vi "Main WT1600.vi"(0 "Settings WT1600 ing":T3={"data bits"=8, "parity"=0, "stop bits"=10, "flow control"=0, "baud rate"=8, "COM"=""} {"baud rate" min=5 max=8 step=1; "flow control" items=["None"=0, "XON/XOFF"=1, "RTS/CTS"=2, "DTR/DSR"=4]; "stop bits" items=["1.0"=10, "1.5"=15, "2.0"=20]; "parity" items=["None", "Odd", "Even", "Mark", "Space"]; "data bits" min=5 max=8 step=1}, 1 "STOP":bool, 2 "Range Tors.":bool, 3 "Numeric":i64, 4 "WT1600 Config ing 3":T1={"Wiring A (0: 1P2W)"=0, "Wiring B (0: 1P2W)"=0, "Wiring C (0: 1P2W)"=0, "V Range (12: 1000)"=12, "V Element (0: All)"=0, "A Element (0: All)"=0, "A Range (9: 5A)"=9, "A Sensor Ratio(mV/A) (10.0000) "=10.0, "Zero Cross Filter (0: OFF)"=0, "Line Filter (0: OFF)"=0, "PT Ratio (1.0000)"=1.0, "Scaling (F: OFF)"=FALSE, "CT Ratio (1.0000)"=1.0, "Scaling Factor (1.0000)"=1.0, "Filter Element (0: All)"=0, "Display Format (0: Numeric)"=0, "Normal Item Amount (1: 4)"=1, "Harmonics Item Amount (1: 4)"=1, "Average Type (0: OFF)"=0, "Average Count (2: 8)"=2, "A Range (9: 5A) 2"=9, "A Sensor Ratio(mV/A) (10.0000)  2"=10.0, "Zero Cross Filter (0: OFF) 2"=0, "Line Filter (0: OFF) 2"=0, "PT Ratio (1.0000) 2"=1.0, "Scaling (F: OFF) 2"=FALSE, "CT Ratio (1.0000) 2"=1.0, "Scaling Factor (1.0000) 2"=1.0, "CUT OFF FREQ"=0.0} {"Wiring A (0: 1P2W)" items=["1P2W", "1P3W", "3P3W", "3P4W", "3V3A"]; "Wiring B (0: 1P2W)" items=["1P2W", "1P3W", "3P3W", "3P4W", "3V3A", "NONE"]; "Wiring C (0: 1P2W)" items=["1P2W", "1P3W", "3P3W", "3P4W", "3V3A", "NONE"]; "V Range (12: 1000)" items=["AUTO", "1.5", "3", "6", "10", "15", "30", "60", "100", "150", "300", "600", "1000"]; "V Element (0: All)" items=["All", "Element 1", "Element 2", "Element 3", "Element 4", "Element 5", "Element 6"]; "A Element (0: All)" items=["All", "Element 1", "Element 2", "Element 3", "Element 4", "Element 5", "Element 6"]; "A Range (9: 5A)" items=["AUTO", "10 mA", "20 mA", "50 mA", "100 mA", "200 mA", "500 mA", "1 A", "2 A", "5 A", "10 A", "20 A", "50 A", "S-AUTO", "50 mV", "100 mV", "250 mV", "500 mV", "1 V", "2.5 V", "5 V", "10 V"]; "Zero Cross Filter (0: OFF)" items=["OFF", "500Hz"]; "Line Filter (0: OFF)" items=["OFF", "500Hz", "5.5kHz"]; "Filter Element (0: All)" items=["All", "Element 1", "Element 2", "Element 3", "Element 4", "Element 5", "Element 6"]; "Display Format (0: Numeric)" items=["Numeric", "Wave", "Bar", "Vector", "Trend", "Numeric & Wave", "Numeric & Bar", "Numeric & Trend", "Wave & Bar", "Wave & Trend", "Bar & Trend", "Information"]; "Normal Item Amount (1: 4)" items=["ALL", "4", "8", "16", "42", "78"]; "Harmonics Item Amount (1: 4)" items=["-", "4", "8", "16", "Single List", "Dual List", "Sigma List"]; "Average Type (0: OFF)" items=["OFF", "Linear", "Exponent"]; "Average Count (2: 8)" items=["2", "4", "8", "16", "32", "64", "128", "256"]; "A Range (9: 5A) 2" items=["AUTO", "10 mA", "20 mA", "50 mA", "100 mA", "200 mA", "500 mA", "1 A", "2 A", "5 A", "10 A", "20 A", "50 A", "S-AUTO", "50 mV", "100 mV", "250 mV", "500 mV", "1 V", "2.5 V", "5 V", "10 V"]; "Zero Cross Filter (0: OFF) 2" items=["OFF", "500Hz"]; "Line Filter (0: OFF) 2" items=["OFF", "500Hz", "5.5kHz"]}, 5 "Refresh":bool, 7 "Path":string) -> (9 "error out":errorcluster, 10 "WT1600 Config ing":T1={"Wiring A (0: 1P2W)"=0, "Wiring B (0: 1P2W)"=0, "Wiring C (0: 1P2W)"=0, "V Range (12: 1000)"=12, "V Element (0: All)"=0, "A Element (0: All)"=0, "A Range (9: 5A)"=9, "A Sensor Ratio(mV/A) (10.0000) "=10.0, "Zero Cross Filter (0: OFF)"=0, "Line Filter (0: OFF)"=0, "PT Ratio (1.0000)"=1.0, "Scaling (F: OFF)"=FALSE, "CT Ratio (1.0000)"=1.0, "Scaling Factor (1.0000)"=1.0, "Filter Element (0: All)"=0, "Display Format (0: Numeric)"=0, "Normal Item Amount (1: 4)"=1, "Harmonics Item Amount (1: 4)"=1, "Average Type (0: OFF)"=0, "Average Count (2: 8)"=2, "A Range (9: 5A) 2"=9, "A Sensor Ratio(mV/A) (10.0000)  2"=10.0, "Zero Cross Filter (0: OFF) 2"=0, "Line Filter (0: OFF) 2"=0, "PT Ratio (1.0000) 2"=1.0, "Scaling (F: OFF) 2"=FALSE, "CT Ratio (1.0000) 2"=1.0, "Scaling Factor (1.0000) 2"=1.0, "CUT OFF FREQ"=0.0} {"Wiring A (0: 1P2W)" items=["1P2W", "1P3W", "3P3W", "3P4W", "3V3A"]; "Wiring B (0: 1P2W)" items=["1P2W", "1P3W", "3P3W", "3P4W", "3V3A", "NONE"]; "Wiring C (0: 1P2W)" items=["1P2W", "1P3W", "3P3W", "3P4W", "3V3A", "NONE"]; "V Range (12: 1000)" items=["AUTO", "1.5", "3", "6", "10", "15", "30", "60", "100", "150", "300", "600", "1000"]; "V Element (0: All)" items=["All", "Element 1", "Element 2", "Element 3", "Element 4", "Element 5", "Element 6"]; "A Element (0: All)" items=["All", "Element 1", "Element 2", "Element 3", "Element 4", "Element 5", "Element 6"]; "A Range (9: 5A)" items=["AUTO", "10 mA", "20 mA", "50 mA", "100 mA", "200 mA", "500 mA", "1 A", "2 A", "5 A", "10 A", "20 A", "50 A", "S-AUTO", "50 mV", "100 mV", "250 mV", "500 mV", "1 V", "2.5 V", "5 V", "10 V"]; "Zero Cross Filter (0: OFF)" items=["OFF", "500Hz"]; "Line Filter (0: OFF)" items=["OFF", "500Hz", "5.5kHz"]; "Filter Element (0: All)" items=["All", "Element 1", "Element 2", "Element 3", "Element 4", "Element 5", "Element 6"]; "Display Format (0: Numeric)" items=["Numeric", "Wave", "Bar", "Vector", "Trend", "Numeric & Wave", "Numeric & Bar", "Numeric & Trend", "Wave & Bar", "Wave & Trend", "Bar & Trend", "Information"]; "Normal Item Amount (1: 4)" items=["ALL", "4", "8", "16", "42", "78"]; "Harmonics Item Amount (1: 4)" items=["-", "4", "8", "16", "Single List", "Dual List", "Sigma List"]; "Average Type (0: OFF)" items=["OFF", "Linear", "Exponent"]; "Average Count (2: 8)" items=["2", "4", "8", "16", "32", "64", "128", "256"]; "A Range (9: 5A) 2" items=["AUTO", "10 mA", "20 mA", "50 mA", "100 mA", "200 mA", "500 mA", "1 A", "2 A", "5 A", "10 A", "20 A", "50 A", "S-AUTO", "50 mV", "100 mV", "250 mV", "500 mV", "1 V", "2.5 V", "5 V", "10 V"]; "Zero Cross Filter (0: OFF) 2" items=["OFF", "500Hz"]; "Line Filter (0: OFF) 2" items=["OFF", "500Hz", "5.5kHz"]}, 11 "error out 2":errorcluster, 12 "Cluster wt1600":T2, 14 "Settings WT1600 out":T3={"data bits"=8, "parity"=0, "stop bits"=10, "flow control"=0, "baud rate"=8, "COM"=""} {"baud rate" min=5 max=8 step=1; "flow control" items=["None"=0, "XON/XOFF"=1, "RTS/CTS"=2, "DTR/DSR"=4]; "stop bits" items=["1.0"=10, "1.5"=15, "2.0"=20]; "parity" items=["None", "Odd", "Even", "Mark", "Space"]; "data bits" min=5 max=8 step=1}, 15 "WT1600":bool, 16 "Errori WT1600":i64, 17 "Measure Value":sgl[](array[numeric]) format="%^.3e", 18 "Coppia":dbl, 19 "Velocità":dbl)   [LabVIEW 2016]
uses:
  QSM PC EXAMPLE.llb/wt1600 variabili.ctl
panel:
  in  "termination char\n(0xA = '\\n' = LF)":u8=10 format="%.0x"
  in  "MaxErr WT1600":i64
  # "ON\nOFF"
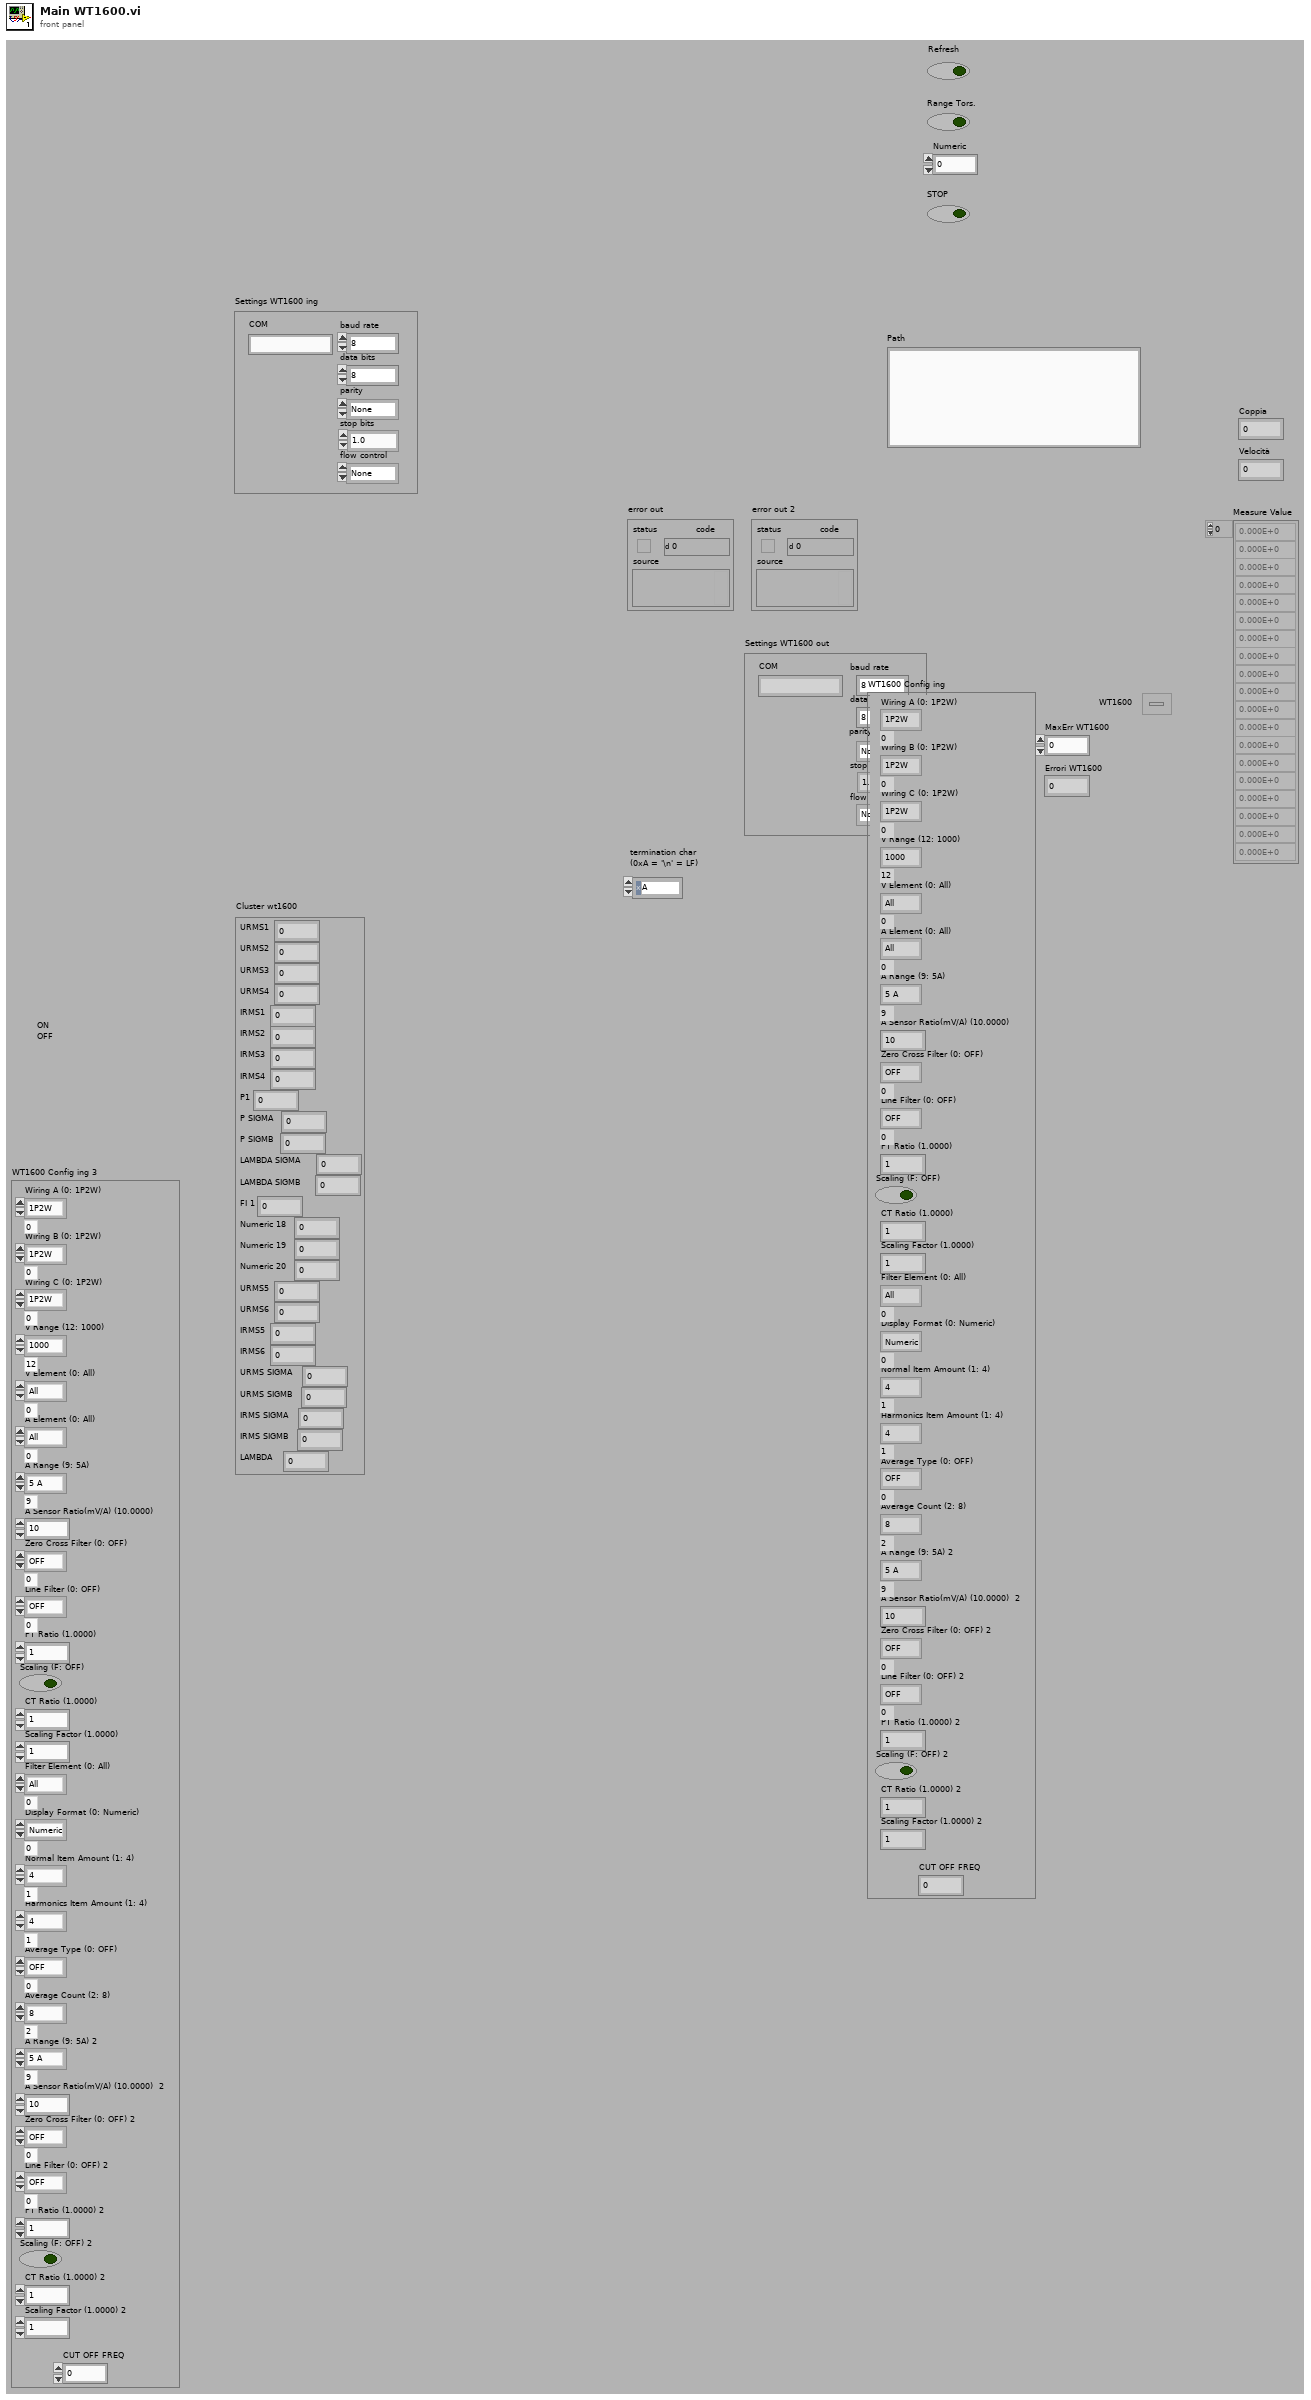
[diagram p1: front panel]
types:
  T1 = cluster{"Wiring A (0: 1P2W)":u16, "Wiring B (0: 1P2W)":u16, "Wiring C (0: 1P2W)":u16, "V Range (12: 1000)":u16, "V Element (0: All)":u16, "A Element (0: All)":u16, "A Range (9: 5A)":u16, "A Sensor Ratio(mV/A) (10.0000) ":dbl, "Zero Cross Filter (0: OFF)":u16, "Line Filter (0: OFF)":u16, "PT Ratio (1.0000)":dbl, "Scaling (F: OFF)":bool, "CT Ratio (1.0000)":dbl, "Scaling Factor (1.0000)":dbl, "Filter Element (0: All)":u16, "Display Format (0: Numeric)":u16, "Normal Item Amount (1: 4)":u16, "Harmonics Item Amount (1: 4)":u16, "Average Type (0: OFF)":u16, "Average Count (2: 8)":u16, "A Range (9: 5A) 2":u16, "A Sensor Ratio(mV/A) (10.0000)  2":dbl, "Zero Cross Filter (0: OFF) 2":u16, "Line Filter (0: OFF) 2":u16, "PT Ratio (1.0000) 2":dbl, "Scaling (F: OFF) 2":bool, "CT Ratio (1.0000) 2":dbl, "Scaling Factor (1.0000) 2":dbl, "CUT OFF FREQ":dbl}
  T2 = typedef "wt1600 variabili.ctl" = cluster{"URMS1":dbl, "URMS2":dbl, "URMS3":dbl, "URMS4":dbl, "IRMS1":dbl, "IRMS2":dbl, "IRMS3":dbl, "IRMS4":dbl, "P1":dbl, "P SIGMA":dbl, "P SIGMB":dbl, "LAMBDA SIGMA":dbl, "LAMBDA SIGMB":dbl, "FI 1":dbl, "Numeric 18":dbl, "Numeric 19":dbl, "Numeric 20":dbl, "URMS5":dbl, "URMS6":dbl, "IRMS5":dbl, "IRMS6":dbl, "URMS SIGMA":dbl, "URMS SIGMB":dbl, "IRMS SIGMA":dbl, "IRMS SIGMB":dbl, "LAMBDA":dbl}
  T3 = cluster{"data bits":u16, "parity":u16, "stop bits":u16, "flow control":u16, "baud rate":u16, "COM":string}
  T4 = cluster{"URMS1":dbl, "URMS2":dbl, "URMS3":dbl, "URMS4":dbl, "IRMS1":dbl, "IRMS2":dbl, "IRMS3":dbl, "IRMS4":dbl, "P1":dbl, "P SIGMA":dbl, "P SIGMB":dbl, "LAMBDA SIGMA":dbl, "LAMBDA SIGMB":dbl, "FI 1":dbl, "Numeric 18":dbl, "Numeric 19":dbl, "Numeric 20":dbl, "URMS5":dbl, "URMS6":dbl, "IRMS5":dbl, "IRMS6":dbl, "URMS SIGMA":dbl, "URMS SIGMB":dbl, "IRMS SIGMA":dbl, "IRMS SIGMB":dbl, "LAMBDA":dbl}
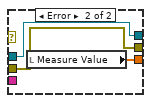
[diagram p4: hidden frame]
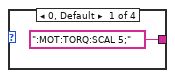
[diagram p6: hidden frame]
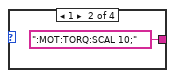
[diagram p7: hidden frame]
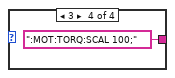
[diagram p8: hidden frame]
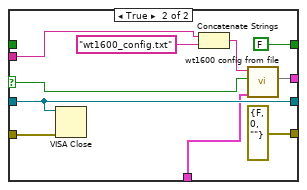
[diagram p10: hidden frame]
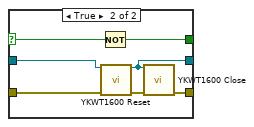
[diagram p13: hidden frame]
diagram:
  n1 = flat-sequence {
    tunnel: [w2] -> w1
    tunnel: w1 -> [w14]
    frame #0 {
      n2 = flat-sequence {
        frame #0 {
        }
      }
      n3 = flat-sequence {
        tunnel: ["Path"] -> w2
        frame #0 {
          n4 = First Call?() -> (First Call?: T/F=w6:bool)
          n5 = case shown="True" w6 {
            tunnel: [w7 w10] -> w4
            tunnel: "Settings WT1600 ing" -> [w7 w11]
            tunnel: "Path" -> [_ w8]
            frame False {
            }
            frame True {
              n6 = local write "MaxErr WT1600"(10) -> ()
              n7 = Concatenate Strings(w8, "wt1600.txt") -> (w12:string)
              n8 = call "Read config COM.vi"("Path"=w12, "Settings WT1600 ing"=w11) -> ("Settings WT1600 out"=w10:T3)  [unwired: 9 out]
            }
          }
          "Settings WT1600 out" <- w4
        }
      }
    }
    frame #1 {
      n9 = while {
        shift-right: [w25] -> _
        shift-left: _ -> [w26]
        shift-right: [w18] -> _
        shift-left: _ -> [w24]
        shift-right: [w19] -> _
        shift-left: _ -> [w27]
        tunnel: w14 -> [w20]
        stop <- TRUE stop-if-true
        n10 = Not(x="STOP") -> (.not. x?=w23:bool)
        n11 = case shown="True" w23 {
          tunnel: w27 -> [_ w81]
          tunnel: w26 -> [w30 w83]
          tunnel: [w30 w91] -> w25
          tunnel: [w31 w90] -> w18
          tunnel: w24 -> [w31 w82]
          tunnel: [FALSE w89] -> w19
          tunnel: w20 -> [_ w72]
          tunnel: [errorcluster {"status"=TRUE, "code"=0, "source"=""} ("´×°oÍ") w34] -> w15
          frame False {
          }
          frame True {
            (unwired) ":NUM:NORM:NUM 8;ITEM1 URMS,SIGMA;ITEM2 IRMS,SIGMA;ITEM3 LAMBDA,SIGMA;ITEM4 FU,1;ITEM5 P,SIGMA;ITEM6 S,SIGMA;ITEM7 Q,SIGMA;ITEM8 IRMS,1; VAL?;"
            # "URMS1\nURMS2\nURMS3\nURMS4\nURMS5\nURMS6\nURMS SIGMA\nURMS SIGMB\nIRMS1\nIRMS2\nIRMS3\nIRMS4\nIRMS5\nIRMS6\nIRMS SIGMA\nIRMS SIGMB\nP1\nP SIGMA\nP SIGMB\nLAMBDA\nLAMBDA SIGMA\nLAMBDA SIGMB\nFI 1"
            n12 = First Call?() -> (First Call?: T/F=w75:bool)
            n13 = Compound Arithmetic op=OR("Refresh", w75) -> (w74:bool)
            n14 = case shown="False" w74 {
              selector: w74 -> [_ w140]
              tunnel: [w134 w145] -> w80
              tunnel: w83 -> [w134 w145]
              tunnel: [w135 errorcluster {"status"=FALSE, "code"=0, "source"=""} ("error out")] -> w79
              tunnel: w82 -> [w135 w144]
              tunnel: [w136 FALSE] -> w78
              tunnel: w81 -> [w136 _]
              tunnel: w72 -> [_ w141]
              tunnel: [w133 w138] -> w33
              tunnel: "WT1600 Config ing 3" -> [w133 w137]
              frame False {
              }
              frame True {
                n15 = VISA Close(VISA resource name=w145, error in (no error)=w144) -> ()  [unwired: 1 out]
                n16 = Concatenate Strings(w141, "wt1600_config.txt") -> (w142:string)
                n17 = call "wt1600 config from file.vi"("WT1600 Config ing"=w137, "leggi"=w140, "Path"=w142) -> (2:w138)  [unwired: 1 in, 7 out]
              }
            }
            "WT1600 Config ing" <- w33
            n18 = case shown="False" w78 {
              tunnel: [w153 w324] -> w71
              tunnel: [w152 w325] -> w35
              tunnel: w79 -> [_ w325]
              tunnel: w80 -> [_ w324]
              tunnel: w33 -> [w155 _]
              frame False {
                w148 = TRUE
                n19 = flat-sequence {
                  tunnel: [TRUE] -> w164
                  tunnel: ["termination char\n(0xA = '\\n' = LF)"] -> w163
                  tunnel: [50] -> w162
                  frame #0 {
                  }
                }
                n20 = local read "Settings WT1600 out"() -> (w161:T3)
                n21 = Unbundle By Name(w161) -> ("COM"=w154:string, "baud rate"=w160:u16, "data bits"=w159:u16, "stop bits"=w158:u16, "flow control"=w156:u16, "parity"=w157:u16)
                n22 = call "OpenCOM.vi"("VISA resource name"=w154, "baud rate (9600)"=w160, "data bits"=w159, "parity"=w157, "stop bits"=w158, "flow control"=w156, "termination char\n(0xA = '\\n' = LF)"=w163, "timeout(ms) solitamente 50ms"=w162, "End Write termination character?"=w164, "End read on termination character?"=w164) -> ("VISA resource name out"=w151:refnum<visa-resource-name>, "error out"=w150:errorcluster)  [unwired: 16 out]
                n23 = call "YKWT1600 Initialize.vi"("VISA session (for class)"=w151, "ID Query (T: Check)"=w148, "Reset (T: Reset)"=w148, "error in (no error)"=w150) -> ("VISA session"=w149:refnum<visa-resource-name>, "error out"=w147:errorcluster)  [unwired: 10 out]
                n24 = case shown="No Error" w147 {
                  tunnel: w155 -> [w167 _]
                  tunnel: w147 -> [w233 w320]
                  tunnel: w149 -> [w232 w319]
                  tunnel: [w230 w319] -> w153
                  tunnel: [w229 w320] -> w152
                  frame No Error {
                    w181 = u16 6 items=["All", "Element 1", "Element 2", "Element 3", "Element 4", "Element 5", "Element 6"] ("Element (0: All)")
                    w180 = u16 5 items=["All", "Element 1", "Element 2", "Element 3", "Element 4", "Element 5", "Element 6"] ("Element (0: All)")
                    w179 = u16 4 items=["All", "Element 1", "Element 2", "Element 3", "Element 4", "Element 5", "Element 6"] ("Element (0: All)")
                    w177 = u16 3 items=["All", "Element 1", "Element 2", "Element 3", "Element 4", "Element 5", "Element 6"] ("Element (0: All)")
                    w178 = u16 2 items=["All", "Element 1", "Element 2", "Element 3", "Element 4", "Element 5", "Element 6"] ("Element (0: All)")
                    w176 = u16 1 items=["All", "Element 1", "Element 2", "Element 3", "Element 4", "Element 5", "Element 6"] ("Element (0: All)")
                    w207 = u16 6 items=["All", "Element 1", "Element 2", "Element 3", "Element 4", "Element 5", "Element 6"] ("Element (0: All)")
                    w208 = u16 5 items=["All", "Element 1", "Element 2", "Element 3", "Element 4", "Element 5", "Element 6"] ("Element (0: All)")
                    w209 = u16 4 items=["All", "Element 1", "Element 2", "Element 3", "Element 4", "Element 5", "Element 6"] ("Element (0: All)")
                    w210 = u16 3 items=["All", "Element 1", "Element 2", "Element 3", "Element 4", "Element 5", "Element 6"] ("Element (0: All)")
                    w206 = u16 2 items=["All", "Element 1", "Element 2", "Element 3", "Element 4", "Element 5", "Element 6"] ("Element (0: All)")
                    w211 = u16 1 items=["All", "Element 1", "Element 2", "Element 3", "Element 4", "Element 5", "Element 6"] ("Element (0: All)")
                    w245 = u16 1 items=["50ms", "100ms", "200ms", "500ms", "1s", "2s", "5s"] ("Update Rate (3: 500ms)")
                    n25 = Unbundle By Name(w167) -> ("Wiring A (0: 1P2W)"=w258:u16, "Wiring B (0: 1P2W)"=w257:u16, "Wiring C (0: 1P2W)"=w256:u16, "V Range (12: 1000)"=w266:u16, "V Element (0: All)"=w265:u16, "A Range (9: 5A)"=w175:u16, "A Sensor Ratio(mV/A) (10.0000)"=w174:dbl, "Zero Cross Filter (0: OFF)"=w203:u16, "Line Filter (0: OFF)"=w204:u16, "PT Ratio (1.0000)"=w202:dbl, "Scaling (F: OFF)"=w205:bool, "CT Ratio (1.0000)"=w201:dbl, "Scaling Factor (1.0000)"=w200:dbl, "Display Format (0: Numeric)"=w264:u16, "Normal Item Amount (1: 4)"=w263:u16, "Harmonics Item Amount (1: 4)"=w262:u16, "Average Type (0: OFF)"=w260:u16, "Average Count (2: 8)"=w259:u16)  [unwired: 2 out]
                    n26 = call "YKWT1600 Config Filter & Scaling.vi"("VISA session"=w232, "Scaling (F: OFF)"=w205, "Element (0: All)"=w211, "Line Filter (0: OFF)"=w204, "WT 1600 Zero Cross Filter (0: OFF)"=w203, "error in (no error)"=w233, "PT Ratio (1.0000)"=w202, "CT Ratio (1.0000)"=w201, "Scaling Factor (1.0000)"=w200) -> ("dup VISA session"=w228:refnum<visa-resource-name>, "error out"=w231:errorcluster)  [unwired: 2 in, 3 out]
                    n27 = flat-sequence {
                      tunnel: w231 -> [w305]
                      tunnel: [w305] -> w227
                      frame #0 {
                        n28 = Wait (ms)(milliseconds to wait=2000) -> ()  [unwired: 1 out]
                      }
                    }
                    n29 = call "YKWT1600 Config Filter & Scaling.vi"("VISA session"=w228, "Scaling (F: OFF)"=w205, "Element (0: All)"=w206, "Line Filter (0: OFF)"=w204, "WT 1600 Zero Cross Filter (0: OFF)"=w203, "error in (no error)"=w227, "PT Ratio (1.0000)"=w202, "CT Ratio (1.0000)"=w201, "Scaling Factor (1.0000)"=w200) -> ("dup VISA session"=w213:refnum<visa-resource-name>, "error out"=w226:errorcluster)  [unwired: 2 in, 3 out]
                    n30 = flat-sequence {
                      tunnel: w226 -> [w303]
                      tunnel: [w303] -> w225
                      frame #0 {
                        n31 = Wait (ms)(milliseconds to wait=2000) -> ()  [unwired: 1 out]
                      }
                    }
                    n32 = call "YKWT1600 Config Filter & Scaling.vi"("VISA session"=w213, "Scaling (F: OFF)"=w205, "Element (0: All)"=w210, "Line Filter (0: OFF)"=w204, "WT 1600 Zero Cross Filter (0: OFF)"=w203, "error in (no error)"=w225, "PT Ratio (1.0000)"=w202, "CT Ratio (1.0000)"=w201, "Scaling Factor (1.0000)"=w200) -> ("dup VISA session"=w216:refnum<visa-resource-name>, "error out"=w224:errorcluster)  [unwired: 2 in, 3 out]
                    n33 = flat-sequence {
                      tunnel: [w300] -> _
                      tunnel: [w300] -> w223
                      tunnel: w224 -> [w300]
                      frame #0 {
                        n34 = Wait (ms)(milliseconds to wait=2000) -> ()  [unwired: 1 out]
                      }
                    }
                    n35 = Unbundle By Name(w167) -> ("Line Filter (0: OFF) 2"=w173:u16, "Zero Cross Filter (0: OFF) 2"=w172:u16, "Scaling (F: OFF) 2"=w171:bool, "PT Ratio (1.0000) 2"=w170:dbl, "CT Ratio (1.0000) 2"=w169:dbl, "Scaling Factor (1.0000) 2"=w168:dbl)
                    n36 = call "YKWT1600 Config Filter & Scaling.vi"("VISA session"=w216, "Scaling (F: OFF)"=w171, "Element (0: All)"=w209, "Line Filter (0: OFF)"=w173, "WT 1600 Zero Cross Filter (0: OFF)"=w172, "error in (no error)"=w223, "PT Ratio (1.0000)"=w170, "CT Ratio (1.0000)"=w169, "Scaling Factor (1.0000)"=w168) -> ("dup VISA session"=w215:refnum<visa-resource-name>, "error out"=w222:errorcluster)  [unwired: 2 in, 3 out]
                    n37 = flat-sequence {
                      tunnel: w222 -> [w299]
                      tunnel: [w299] -> w221
                      frame #0 {
                        n38 = Wait (ms)(milliseconds to wait=2000) -> ()  [unwired: 1 out]
                      }
                    }
                    n39 = call "YKWT1600 Config Filter & Scaling.vi"("VISA session"=w215, "Scaling (F: OFF)"=w171, "Element (0: All)"=w208, "Line Filter (0: OFF)"=w173, "WT 1600 Zero Cross Filter (0: OFF)"=w172, "error in (no error)"=w221, "PT Ratio (1.0000)"=w170, "CT Ratio (1.0000)"=w169, "Scaling Factor (1.0000)"=w168) -> ("dup VISA session"=w214:refnum<visa-resource-name>, "error out"=w220:errorcluster)  [unwired: 2 in, 3 out]
                    n40 = flat-sequence {
                      tunnel: w220 -> [w297]
                      tunnel: [w297] -> w219
                      frame #0 {
                        n41 = Wait (ms)(milliseconds to wait=2000) -> ()  [unwired: 1 out]
                      }
                    }
                    n42 = call "YKWT1600 Config Filter & Scaling.vi"("VISA session"=w214, "Scaling (F: OFF)"=w171, "Element (0: All)"=w207, "Line Filter (0: OFF)"=w173, "WT 1600 Zero Cross Filter (0: OFF)"=w172, "error in (no error)"=w219, "PT Ratio (1.0000)"=w170, "CT Ratio (1.0000)"=w169, "Scaling Factor (1.0000)"=w168) -> ("dup VISA session"=w212:refnum<visa-resource-name>, "error out"=w218:errorcluster)  [unwired: 2 in, 3 out]
                    n43 = flat-sequence {
                      tunnel: w218 -> [w295]
                      tunnel: [w295] -> w217
                      frame #0 {
                        n44 = Wait (ms)(milliseconds to wait=2000) -> ()  [unwired: 1 out]
                      }
                    }
                    n45 = call "YKWT1600 Config Voltage.vi"("VISA session"=w212, "Element (0: All)"=w265, "V Range (12: 1000)"=w266, "error in (no error)"=w217) -> ("dup VISA session"=w268:refnum<visa-resource-name>, "error out"=w267:errorcluster)  [unwired: 10 out]
                    n46 = call "YKWT1600 Config Current.vi"("VISA session"=w268, "Element (0: All)"=w176, "A Range (9: 5A)"=w175, 9:w174, "error in (no error)"=w267) -> ("dup VISA session"=w183:refnum<visa-resource-name>, "error out"=w189:errorcluster)  [unwired: 9 out]
                    n47 = flat-sequence {
                      tunnel: w189 -> [w293]
                      tunnel: [w293] -> w199
                      frame #0 {
                        n48 = Wait (ms)(milliseconds to wait=2000) -> ()  [unwired: 1 out]
                      }
                    }
                    n49 = call "YKWT1600 Config Current.vi"("VISA session"=w183, "Element (0: All)"=w178, "A Range (9: 5A)"=w175, 9:w174, "error in (no error)"=w199) -> ("dup VISA session"=w187:refnum<visa-resource-name>, "error out"=w198:errorcluster)  [unwired: 9 out]
                    n50 = flat-sequence {
                      tunnel: w198 -> [w291]
                      tunnel: [w291] -> w197
                      frame #0 {
                        n51 = Wait (ms)(milliseconds to wait=2000) -> ()  [unwired: 1 out]
                      }
                    }
                    n52 = call "YKWT1600 Config Current.vi"("VISA session"=w187, "Element (0: All)"=w177, "A Range (9: 5A)"=w175, 9:w174, "error in (no error)"=w197) -> ("dup VISA session"=w186:refnum<visa-resource-name>, "error out"=w196:errorcluster)  [unwired: 9 out]
                    n53 = flat-sequence {
                      tunnel: w196 -> [w289]
                      tunnel: [w289] -> w195
                      frame #0 {
                        n54 = Wait (ms)(milliseconds to wait=2000) -> ()  [unwired: 1 out]
                      }
                    }
                    n55 = Unbundle By Name(w167) -> ("A Range (9: 5A) 2"=w166:u16, "A Sensor Ratio(mV/A) (10.0000)  2"=w165:dbl)
                    n56 = call "YKWT1600 Config Current.vi"("VISA session"=w186, "Element (0: All)"=w179, "A Range (9: 5A)"=w166, 9:w165, "error in (no error)"=w195) -> ("dup VISA session"=w185:refnum<visa-resource-name>, "error out"=w194:errorcluster)  [unwired: 9 out]
                    n57 = flat-sequence {
                      tunnel: w194 -> [w287]
                      tunnel: [w287] -> w193
                      frame #0 {
                        n58 = Wait (ms)(milliseconds to wait=2000) -> ()  [unwired: 1 out]
                      }
                    }
                    n59 = call "YKWT1600 Config Current.vi"("VISA session"=w185, "Element (0: All)"=w180, "A Range (9: 5A)"=w166, 9:w165, "error in (no error)"=w193) -> ("dup VISA session"=w184:refnum<visa-resource-name>, "error out"=w192:errorcluster)  [unwired: 9 out]
                    n60 = flat-sequence {
                      tunnel: [w284] -> w191
                      tunnel: w192 -> [w284]
                      frame #0 {
                        n61 = Wait (ms)(milliseconds to wait=2000) -> ()  [unwired: 1 out]
                      }
                    }
                    n62 = call "YKWT1600 Config Current.vi"("VISA session"=w184, "Element (0: All)"=w181, "A Range (9: 5A)"=w166, 9:w165, "error in (no error)"=w191) -> ("dup VISA session"=w182:refnum<visa-resource-name>, "error out"=w190:errorcluster)  [unwired: 9 out]
                    n63 = flat-sequence {
                      tunnel: [w282] -> w188
                      tunnel: w190 -> [w282]
                      frame #0 {
                        n64 = Wait (ms)(milliseconds to wait=2000) -> ()  [unwired: 1 out]
                      }
                    }
                    n65 = call "YKWT1600 Config Display Format.vi"("VISA session"=w182, "Display Format (0: Numeric)"=w264, "Normal Item Amount (1: 4)"=w263, "Harmonics Item Amount (1: 4)"=w262, "error in (no error)"=w188) -> ("dup VISA session"=w249:refnum<visa-resource-name>, "error out"=w250:errorcluster)  [unwired: 9 out]
                    n66 = flat-sequence {
                      tunnel: w250 -> [w316]
                      tunnel: [w316] -> w247
                      frame #0 {
                        n67 = Wait (ms)(milliseconds to wait=2000) -> ()  [unwired: 1 out]
                      }
                    }
                    n68 = call "YKWT1600 Config Update Rate.vi"("VISA session"=w249, "Update Rate (3: 500ms)"=w245, "error in (no error)"=w247) -> ("dup VISA session"=w248:refnum<visa-resource-name>, "error out"=w246:errorcluster)  [unwired: 11 out]
                    n69 = flat-sequence {
                      tunnel: [w274] -> w261
                      tunnel: [w275] -> w235
                      tunnel: w248 -> [w273]
                      tunnel: w246 -> [w272]
                      tunnel: w256 -> [w269]
                      tunnel: w257 -> [w270]
                      tunnel: w258 -> [w271]
                      frame #0 {
                        n70 = call "YKWT1600 Config Wiring.vi"("VISA session"=w273, "Wiring A (0: 1P2W)"=w271, "Wiring B (0: 1P2W)"=w270, "Wiring C (0: 1P2W)"=w269, "error in (no error)"=w272) -> ("dup VISA session"=w274:refnum<visa-resource-name>, "error out"=w275:errorcluster)  [unwired: 9 out]
                      }
                    }
                    n71 = flat-sequence {
                      tunnel: w235 -> [w306]
                      tunnel: [w306] -> w234
                      frame #0 {
                        n72 = Wait (ms)(milliseconds to wait=2000) -> ()  [unwired: 1 out]
                      }
                    }
                    n73 = flat-sequence {
                      tunnel: w261 -> [w281]
                      tunnel: [w280] -> w255
                      tunnel: w234 -> [w279]
                      tunnel: [w278] -> w237
                      tunnel: w260 -> [w277]
                      tunnel: w259 -> [w276]
                      frame #0 {
                        n74 = call "YKWT1600 Config Measure Average.vi"("VISA session"=w281, "Average Type (0: OFF)"=w277, "Average Count (2: 8)"=w276, "error in (no error)"=w279) -> ("dup VISA session"=w280:refnum<visa-resource-name>, "error out"=w278:errorcluster)  [unwired: 10 out]
                      }
                    }
                    n75 = flat-sequence {
                      tunnel: w237 -> [w309]
                      tunnel: [w309] -> w236
                      frame #0 {
                        n76 = Wait (ms)(milliseconds to wait=2000) -> ()  [unwired: 1 out]
                      }
                    }
                    n77 = VISA Write(VISA resource name=w255, write buffer=":MOT:FILT:LINE 100;", error in (no error)=w236) -> (VISA resource name out=w238:refnum<visa-resource-name>, error out=w252:errorcluster)  [unwired: 1 out]
                    n78 = flat-sequence {
                      tunnel: w252 -> [w318]
                      tunnel: [w318] -> w251
                      frame #0 {
                        n79 = Wait (ms)(milliseconds to wait=2000) -> ()  [unwired: 1 out]
                      }
                    }
                    n80 = VISA Write(VISA resource name=w238, write buffer=":MOT:SPE:RANG 10V;:MOT:TORQ:RANG 10V;", error in (no error)=w251) -> (VISA resource name out=w240:refnum<visa-resource-name>, error out=w244:errorcluster)  [unwired: 1 out]
                    n81 = flat-sequence {
                      tunnel: w244 -> [w313]
                      tunnel: [w313] -> w242
                      tunnel: w240 -> [w314]
                      tunnel: [w314] -> w239
                      frame #0 {
                        n82 = Wait (ms)(milliseconds to wait=2000) -> ()  [unwired: 1 out]
                      }
                    }
                    n83 = VISA Write(VISA resource name=w239, write buffer=":MOT:SPE:SCAL 500;:MOT:TORQ:SCAL 5;", error in (no error)=w242) -> (VISA resource name out=w230:refnum<visa-resource-name>, error out=w241:errorcluster)  [unwired: 1 out]
                    n84 = flat-sequence {
                      tunnel: w241 -> [w311]
                      tunnel: [w311] -> w229
                      frame #0 {
                        n85 = Wait (ms)(milliseconds to wait=2000) -> ()  [unwired: 1 out]
                      }
                    }
                    "error out" <- w233
                    "error out 2" <- w217
                  }
                  frame Error {
                  }
                }
              }
              frame True {
              }
            }
            n86 = case shown="True" "Range Tors." {
              tunnel: w71 -> [w102 w110]
              tunnel: w35 -> [w101 w109]
              tunnel: [w101 w108] -> w40
              tunnel: [w102 w107] -> w69
              frame False {
              }
              frame True {
                n87 = case shown="2" "Numeric" {
                  tunnel: [":MOT:TORQ:SCAL 5;" ":MOT:TORQ:SCAL 10;" ":MOT:TORQ:SCAL 50;" ":MOT:TORQ:SCAL 100;"] -> w104
                  frame 0, Default {
                  }
                  frame 1 {
                  }
                  frame 2 {
                  }
                  frame 3 {
                  }
                }
                n88 = flat-sequence {
                  tunnel: w104 -> [w119]
                  tunnel: w110 -> [w118]
                  tunnel: w109 -> [w117]
                  tunnel: [w116] -> w106
                  tunnel: [w115] -> w105
                  tunnel: [w121] -> w107
                  tunnel: [w122] -> w108
                  tunnel: w106 -> [w122]
                  tunnel: w105 -> [w121]
                  frame #0 {
                    n89 = VISA Write(VISA resource name=w118, write buffer=w119, error in (no error)=w117) -> (VISA resource name out=w115:refnum<visa-resource-name>, error out=w116:errorcluster)  [unwired: 1 out]
                  }
                  frame #1 {
                    n90 = Wait (ms)(milliseconds to wait=2000) -> ()  [unwired: 1 out]
                  }
                }
              }
            }
            n91 = case shown="No Error" w40 {
              tunnel: w40 -> [w97 w99]
              tunnel: w69 -> [w96 w100]
              tunnel: ":NUM:NORM:NUM 25;ITEM1 URMS,1;ITEM2 URMS,2;ITEM3 URMS,3;ITEM4 URMS,4;ITEM5 URMS,5;ITEM6 URMS,6;ITEM7 URMS,SIGMA;ITEM8 URMS,SIGMB;ITEM9 IRMS,1;ITEM10 IRMS,2;ITEM11 IRMS,3;ITEM12 IRMS,4;ITEM13 IRMS,5;ITEM14 IRMS,6;ITEM15 IRMS,SIGMA;ITEM16 IRMS,SIGMB;ITEM17 P,1;ITEM18 P,SIGMA;ITEM19 P,SIGMB;ITEM20 LAMBDA,1;ITEM21 LAMBDA,SIGMA;ITEM22 LAMBDA,SIGMB;ITEM23 FU,1;ITEM24 TORQ;ITEM25 SPE;VAL?;" -> [w95 _]
              tunnel: [w94 w99] -> w39
              tunnel: [w93 w100] -> w67
              tunnel: [w92 w98] -> w51
              frame No Error {
                n92 = call "WT1600(Read Array).vi"("Read"=w95, "error in (no error)"=w97, "VISA session"=w96) -> ("error out"=w94:errorcluster, "Measure 2"=w92:dbl[], "dup VISA session"=w93:refnum<visa-resource-name>)  [unwired: 6 out]
              }
              frame Error {
                n93 = local read "Measure Value"() -> (w98:sgl[])
              }
            }
            "Measure Value" <- w51
            n94 = case shown="True" FALSE {
              tunnel: w67 -> [w124 w128]
              tunnel: w39 -> [w123 w127]
              tunnel: [w123 w132] -> w34
              tunnel: [w124 w131] -> w77
              frame False {
              }
              frame True {
                n95 = call "WT1600(Read Array).vi"("Read"=":NUM:NORM:NUM 2;ITEM1 TORQ;ITEM2 SPE;VAL?;", "error in (no error)"=w127, "VISA session"=w128) -> ("error out"=w132:errorcluster, "Measure 2"=w130:dbl[], "dup VISA session"=w131:refnum<visa-resource-name>)  [unwired: 6 out]
                n96 = Index Array(array=w130) -> (element #1=→"Coppia":dbl, element #2=→"Velocità":dbl)  [unwired: 2 in]
              }
            }
            n97 = Index Array(array=w51) -> (element #1=w65:dbl, element #2=w64:dbl, element #3=w63:dbl, element #4=w62:dbl, element #5=w61:dbl, element #6=w60:dbl, element #7=w59:dbl, element #8=w58:dbl, element #9=w57:dbl, element #10=w56:dbl, element #11=w55:dbl, element #12=w54:dbl, element #13=w53:dbl, element #14=w52:dbl, element #15=w50:dbl, element #16=w49:dbl, element #17=w48:dbl, element #18=w47:dbl, element #19=w46:dbl, element #20=w45:dbl, element #21=w44:dbl, element #22=w43:dbl, element #23=w42:dbl, element #24=w37:dbl, element #25=w36:dbl)  [unwired: 25 in]
            n98 = Bundle By Name(cluster=T4 {"URMS1"=0.0, "URMS2"=0.0, "URMS3"=0.0, "URMS4"=0.0, "IRMS1"=0.0, "IRMS2"=0.0, "IRMS3"=0.0, "IRMS4"=0.0, "P1"=0.0, "P SIGMA"=0.0, "P SIGMB"=0.0, "LAMBDA SIGMA"=0.0, "LAMBDA SIGMB"=0.0, "FI 1"=0.0, "Numeric 18"=0.0, "Numeric 19"=0.0, "Numeric 20"=0.0, "URMS5"=0.0, "URMS6"=0.0, "IRMS5"=0.0, "IRMS6"=0.0, "URMS SIGMA"=0.0, "URMS SIGMB"=0.0, "IRMS SIGMA"=0.0, "IRMS SIGMB"=0.0, "LAMBDA"=0.0} ("Cluster wt1600"), "URMS1"=w65, "URMS2"=w64, "URMS3"=w63, "URMS4"=w62, "URMS5"=w61, "URMS6"=w60, "URMS SIGMA"=w59, "URMS SIGMB"=w58, "IRMS1"=w57, "IRMS2"=w56, "IRMS3"=w55, "IRMS4"=w54, "IRMS5"=w53, "IRMS6"=w52, "IRMS SIGMA"=w50, "IRMS SIGMB"=w49, "P1"=w48, "P SIGMA"=w47, "P SIGMB"=w46, "LAMBDA"=w45, "LAMBDA SIGMA"=w44, "LAMBDA SIGMB"=w43, "FI 1"=w42) -> (→"Cluster wt1600":T4)
            n99 = local write "Coppia"(w37) -> ()
            n100 = local write "Velocità"(w36) -> ()
            n101 = local read "Errori WT1600"() -> (w86:i64)
            n102 = call "Com Errori.vi"("VISA session"=w77, "Errori in"=w86, "Max Errori"="MaxErr WT1600", "error in (no error)"=w34) -> ("dup VISA session"=w88:refnum<visa-resource-name>, "Errori out"=w85:i64, "Chiudi com"=w70:bool, "error out"=w87:errorcluster)  [unwired: 20 out]
            n103 = local write "Errori WT1600"(w85) -> ()
            n104 = case shown="False" w70 {
              selector: w70 -> [_ w335]
              tunnel: w87 -> [w327 w329]
              tunnel: w88 -> [w328 w332]
              tunnel: [w327 w333] -> w90
              tunnel: [w328 w331] -> w91
              tunnel: [TRUE w334] -> w89
              frame False {
              }
              frame True {
                n105 = Not(x=w335) -> (.not. x?=w334:bool)
                n106 = call "YKWT1600 Reset.vi"("VISA session"=w332, "error in (no error)"=w329) -> ("dup VISA session"=w331:refnum<visa-resource-name>, "error out"=w330:errorcluster)  [unwired: 12 out]
                n107 = call "YKWT1600 Close.vi"("VISA session"=w331, "error in (no error)"=w330) -> ("error out"=w333:errorcluster)  [unwired: 13 out]
              }
            }
          }
        }
        n108 = Unbundle By Name(w15) -> ("status"=w17:bool)
        n109 = Not(x=w17) -> (.not. x?=→"WT1600":bool)
      }
    }
  }
